vi "repmat (dbl 1d).vi"(7 "orientation":enum16{"row", "column"}(ring), 9 "c":i32=1, 10 "r":i32=1, 11 "array in":dbl[](array[numeric])) -> (3 "array out":dbl[](array[numeric]))   [LabVIEW 2012, in "common.lvlib"]
uses:
  common.lvlib
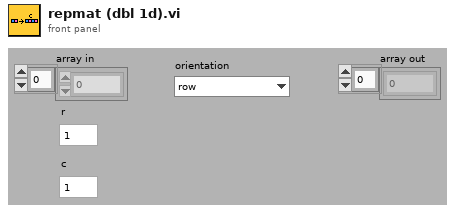
[diagram p1: front panel]
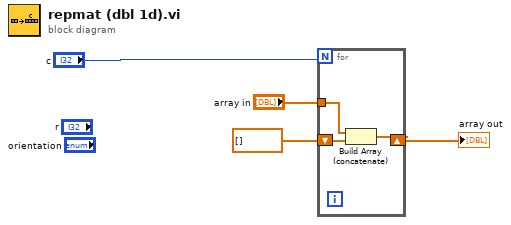
[diagram p0: block diagram]
diagram:
  n1 = for {
    N: "c" -> [_]
    tunnel: "array in" -> [w6]
    shift-right: [w5] -> w1
    shift-left: dbl[] [] ("vector") -> [w7]
    n2 = Build Array (concatenate)(w6, w7) -> (w5:dbl[])
  }
  "array out" <- w1
